vi "SshKeywordWrite.vi"(0 "error in (no error)":errorcluster, 1 "Pattern":string, 5 "Value":string, 6 "SshStream in":refnum<k24>, 7 "Service":string, 9 "Keyword":string) -> (2 "Result":string, 3 "error out":errorcluster, 10 "SshStream out":refnum<k24>)   [LabVIEW 2009]
uses:
  C:/Ohana/LV2009/OhanaOS-LV81/Instruments/Keyword/Controller/Tamir.sharpSsh.dll
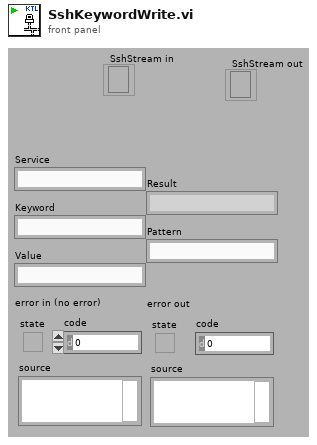
[diagram p1: front panel]
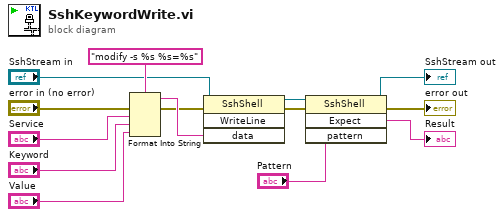
[diagram p0: block diagram]
diagram:
  n1 = Format Into String(format string="modify -s %s %s=%s" ("data"), error in="error in (no error)", "Service", "Keyword", "Value") -> (resulting string=w14:string, error out=w12:errorcluster)  [unwired: 1 in]
  n2 = invoke class="SshShell" method="WriteLine"(reference="SshStream in", error in=w12, "data"=w14) -> (reference out=w8:refnum<k24>, error out=w9:errorcluster)  [unwired: 1 in, 2 out]
  n3 = invoke class="SshShell" method="Expect"(reference=w8, error in=w9, "pattern"="Pattern") -> (reference out=→"SshStream out":refnum<k24>, error out=→"error out":errorcluster, "Expect"=→"Result":string)  [unwired: 1 in, 1 out]
